vi "Initialize.vi"(8 "Error In":errorcluster, 11 "VI Path":path) -> (0 "Error Out":errorcluster, 2 "Action Queues":T1, 3 "Executable Configuration":T2)   [LabVIEW 2012]
uses:
  ExecutableConfiguration.ctl
  ActionQueues.ctl
  UIActionQueueElement.ctl
  UIAction.ctl
  HardwareActionQueueElement.ctl
  HardwareAction.ctl
  libs/LV-Utilities/LV-Utilities.lvlib
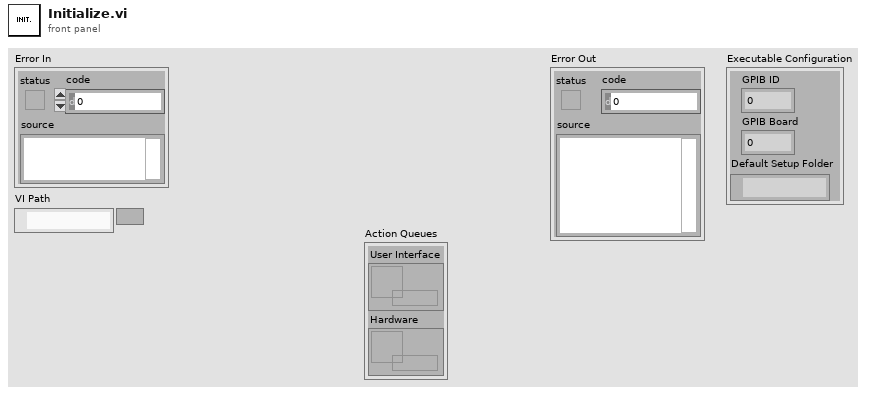
[diagram p1: front panel]
types:
  T1 = typedef "ActionQueues.ctl" = cluster{"User Interface":refnum<queue>, "Hardware":refnum<queue>}
  T2 = typedef "ExecutableConfiguration.ctl" = cluster{"GPIB ID":u8, "GPIB Board":u8, "Default Setup Folder":path}
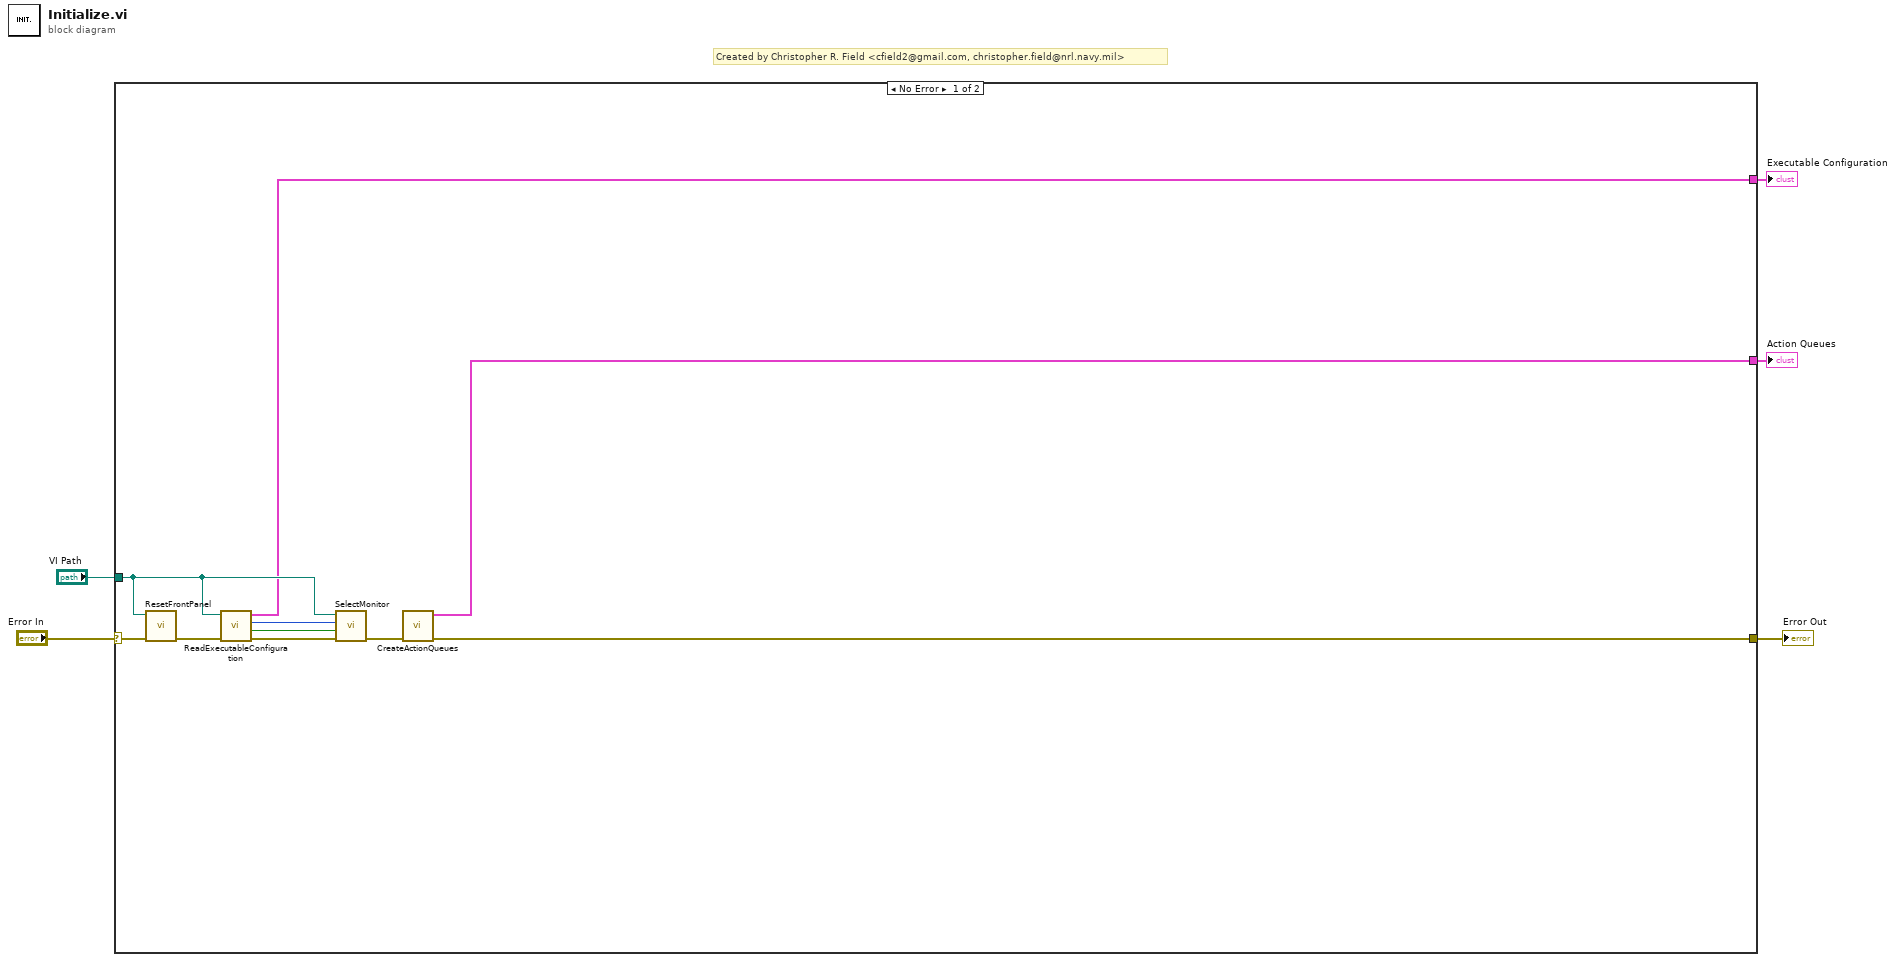
[diagram p0: block diagram]
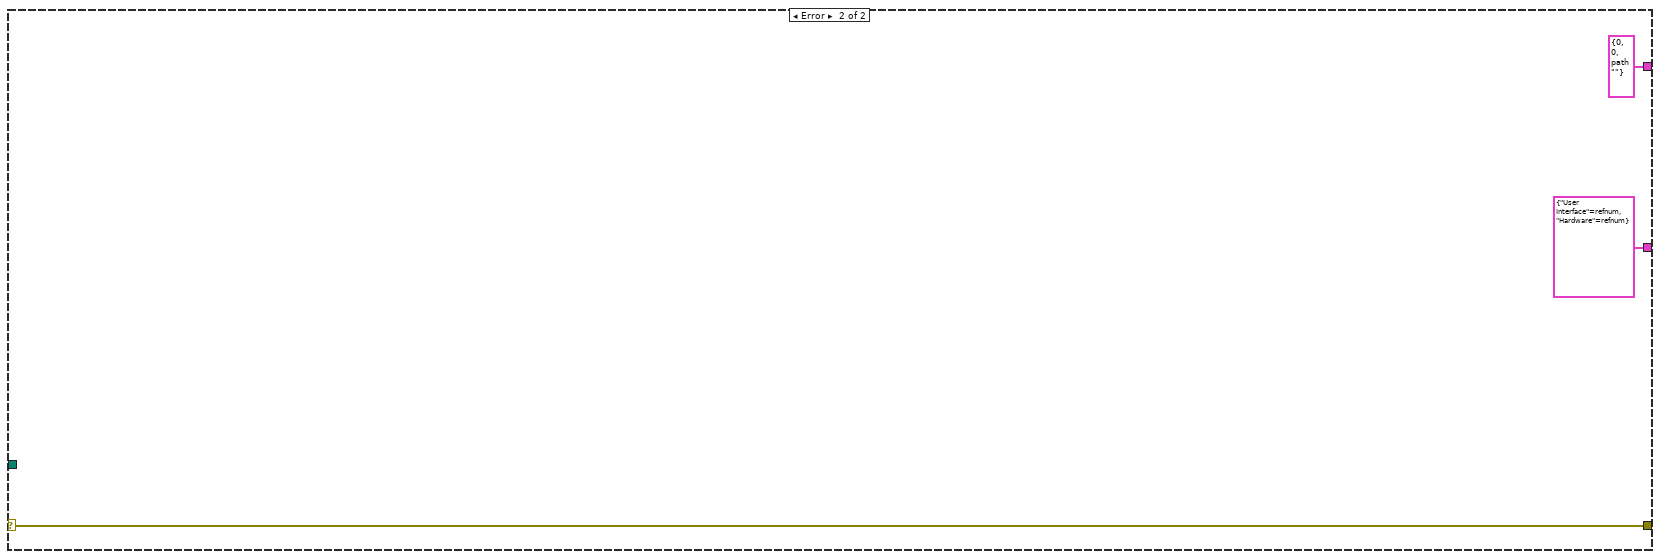
[diagram p2: hidden frame]
diagram:
  # "Created by Christopher R. Field <cfield2@gmail.com, christopher.field@nrl.navy.mil>"
  n1 = case shown="No Error" "Error In" {
    selector: "Error In" -> [w15 w18]
    tunnel: "VI Path" -> [w10 _]
    tunnel: [w7 w18] -> w3
    tunnel: [w9 T2 {"GPIB ID"=0, "GPIB Board"=0, "Default Setup Folder"=path ""} ("Executable Configuration")] -> w2
    tunnel: [w6 T1 {"User Interface"=refnum, "Hardware"=refnum} ("Action Queues")] -> w1
    frame No Error {
      n2 = call "ResetFrontPanel.vi"("Error In"=w15, "VI Path"=w10) -> ("Error Out"=w14:errorcluster)  [unwired: 9 in]
      n3 = call "ReadExecutableConfiguration.vi"("Error In"=w14, "VI Path"=w10) -> ("Error Out"=w12:errorcluster, "Center On Monitor?"=w11:bool, "Monitor (0 = primary)"=w13:i32, "Executable Configuration"=w9:T2)  [unwired: 6 in]
      n4 = call "SelectMonitor.vi"("Error In"=w12, "Center?"=w11, "Monitor (0=primary)"=w13, "VI Path"=w10) -> ("Error out"=w8:errorcluster)  [unwired: 7 in]
      n5 = call "CreateActionQueues.vi"("Error In"=w8) -> ("Error Out"=w7:errorcluster, "Action Queues"=w6:T1)  [unwired: 9 in]
    }
    frame Error {
    }
  }
  "Error Out" <- w3
  "Executable Configuration" <- w2
  "Action Queues" <- w1
